vi "Serial Debug.vi"() -> ()   [LabVIEW 2018]
uses:
  <vilib>/Rock Robotics/SystemInterfaces/spilib/spi_bus.ctl
  source/library/Interface/Pixy Com.lvclass
  source/deviceSupport/FRC/SPI/RoboRIO SPI.lvclass
  source/deviceSupport/FRC/UART/RoboRIO UART.lvclass
  <vilib>/Rock Robotics/WPI/SerialPort/WPI_SerialPort.ctl
panel:
  out "header":u8[](array[numeric])
  out "error out":errorcluster
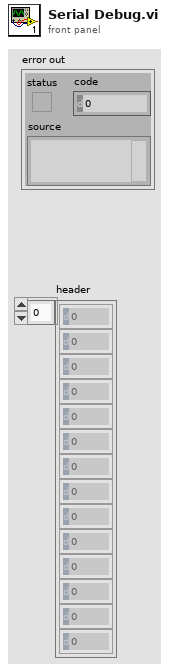
[diagram p1: front panel]
types:
  T1 = typedef "spi_bus.ctl" = enum16{"SPI On-Board, CS0", "SPI On-Board, CS1", "SPI On-Board, CS2", "SPI On-Board, CS3", "SPI MXP", "Invalid"}
  T2 = typedef "WPI_SerialPort.ctl" = enum16{"Onboard RS-232", "MXP TTL", "USB 1", "USB 2"}
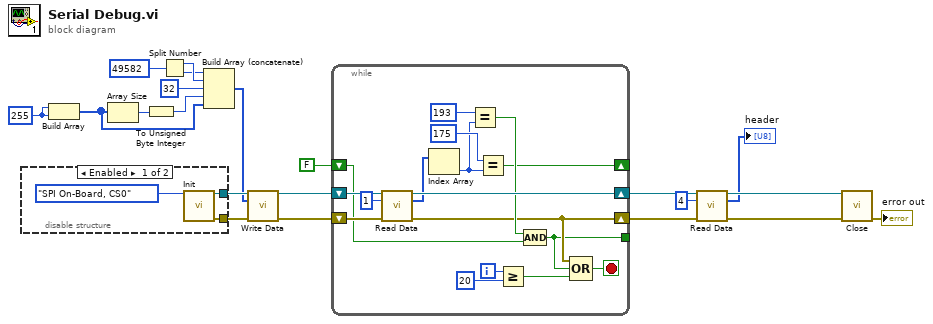
[diagram p0: block diagram]
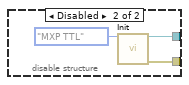
[diagram p2: hidden frame]
diagram:
  w21 = u8 255 ("signature map")
  n1 = disable-structure shown="Enabled" {
    disable-tunnel: [w23 w26] -> w14
    disable-tunnel: [w22 w27] -> w13
    frame Enabled {
      n2 = call "Init.vi"("SPI Bus"=spi_bus."SPI On-Board, CS0") -> ("comm interface out"=w22:refnum<class "Pixy Com.lvclass">, "error out"=w23:errorcluster)  [unwired: 13 in]
    }
    frame Disabled {
      n3 = call "Init.vi"("serial port"=WPI_SerialPort."MXP TTL") -> ("comm interface out"=w27:refnum<class "Pixy Com.lvclass">, "error out"=w26:errorcluster)  [unwired: 13 in]
    }
  }
  n4 = Build Array(w21, w21) -> (w11:u8[])
  n5 = Array Size(array=w11) -> (size(s)=w15:i32)
  n6 = To Unsigned Byte Integer(number=w15) -> (unsigned 8bit integer=w16:u8)
  n7 = Split Number(x=u16 49582) -> (hi(x)=w18:u8, lo(x)=w17:u8)
  n8 = Build Array (concatenate)(w17, w18, u8 32 ("element"), w16, w11) -> (w10:u8[])
  n9 = call-dynamic "Write Data.vi"("comm interface in"=w13, "data"=w10, "error in"=w14) -> ("comm interface out"=w9:refnum<class "Pixy Com.lvclass">, "error out"=w8:errorcluster)  [unwired: 11 in]
  n10 = while {
    shift-right: [w42] -> w4
    shift-left: w9 -> [w44]
    shift-right: [w34] -> w5
    shift-left: w8 -> [w43]
    shift-right: [w35] -> _
    shift-left: FALSE -> [w30]
    tunnel: [w29] -> _
    i -> [w33]
    stop <- w31 stop-if-true
    n11 = call-dynamic "Read Data.vi"("comm interface in"=w44, "bytes to read"=1, "error in"=w43) -> ("comm interface out"=w42:refnum<class "Pixy Com.lvclass">, "data"=w40:u8[], "error out"=w34:errorcluster)  [unwired: 10 in]
    n12 = Index Array(array=w40) -> (element=w38:u8)  [unwired: 1 in]
    n13 = Equal?(x=u8 193 ("element"), y=w38) -> (x = y?=w36:bool)
    n14 = Equal?(x=u8 175 ("element"), y=w38) -> (x = y?=w35:bool)
    n15 = Greater Or Equal?(x=w33, y=20 ("signature map")) -> (x >= y?=w32:bool)
    n16 = Compound Arithmetic op=AND(w36, w30) -> (w29:bool)
    n17 = Compound Arithmetic op=OR(w34, w29, w32) -> (w31:bool)
  }
  n18 = call-dynamic "Read Data.vi"("comm interface in"=w4, "bytes to read"=4, "error in"=w5) -> ("comm interface out"=w2:refnum<class "Pixy Com.lvclass">, "data"=→"header":u8[], "error out"=w3:errorcluster)  [unwired: 10 in]
  n19 = call-dynamic "Close.vi"("comm interface in"=w2, "error in"=w3) -> ("error out"=→"error out":errorcluster)  [unwired: 13 in]
